vi "ZK固件状态读取.vi"(7 "是否启用通讯通知":bool, 8 "error in (no error)":errorcluster, 11 "Slave ID":T2) -> (0 "error out":errorcluster, 3 "固件状态":T1 items=["砖头"=0, "APP正常"=65535])   [LabVIEW 2016, in "质控单元V4.lvlib"]
uses:
  <vilib>/Plasmionique/MB Master/MB_Master/MB_Master.lvclass
  <vilib>/Plasmionique/MB Master/MB Master.lvlib
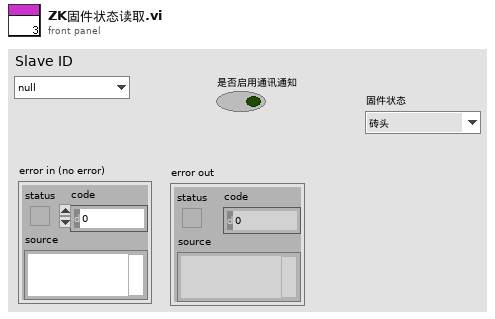
[diagram p1: front panel]
types:
  T1 = typedef "质控单元V4.lvlib/固件状态.ctl" = u16
  T2 = typedef "质控单元V4.lvlib/质控slave id.ctl" = enum16{"null", "氨氮", "总磷", "总氮", "CODMn", "CODCr"}
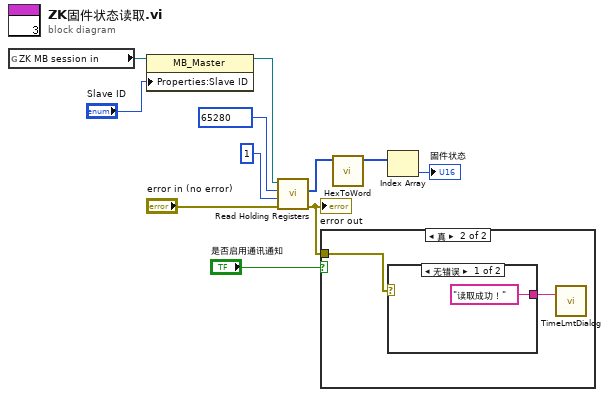
[diagram p0: block diagram]
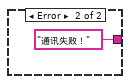
[diagram p3: hidden frame]
diagram:
  n1 = global read "ZK非断电保存全局变量.vi" "ZK MB session in"() -> (w10:refnum<class "MB_Master.lvclass">)
  n2 = property class="MB_Master"(reference=w10, "Properties:Slave ID"="Slave ID") -> (reference out=w8:refnum<class "MB_Master.lvclass">)  [unwired: 1 in, 1 out]
  n3 = call <vilib>:"Read Holding Registers.vi"("error in (no error)"="error in (no error)", "quantity"=u16 1, "starting address"=u16 65280, "MB session in"=w8) -> ("error out"=w2:errorcluster, "Registers"=w5:u16[])  [unwired: 5 in, 1 out]
  "error out" <- w2
  n4 = case shown="真" "是否启用通讯通知" {
    tunnel: w2 -> [_ w13]
    frame False {
    }
    frame True {
      n5 = case shown="无错误" w13 {
        tunnel: ["读取成功！" "通讯失败！"] -> w12
        frame No Error {
        }
        frame Error {
        }
      }
      n6 = call "TimeLmtDialog.vi"("Infoin"=w12) -> ()  [unwired: 11 in]
    }
  }
  n7 = call "HexToWord.vi"("数组"=w5) -> ("WORD"=w4:u16[])  [unwired: 10 in]
  n8 = Index Array(array=w4) -> (element=→"固件状态":u16)  [unwired: 1 in]
